vi "GetSystemSerialNumber.vi"(0 "VISA resource name":refnum<visa-resource-name>="COM5", 11 "error in (no error)":errorcluster, 12 "Open Serial":bool, 14 "Close Serial":bool) -> (3 "S/N":string="0", 4 "VISA resource name out":refnum<visa-resource-name>="COM5", 15 "error out":errorcluster)   [LabVIEW 2018]
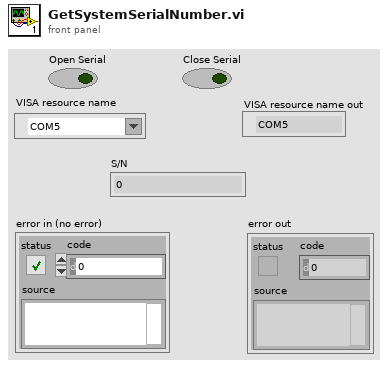
[diagram p1: front panel]
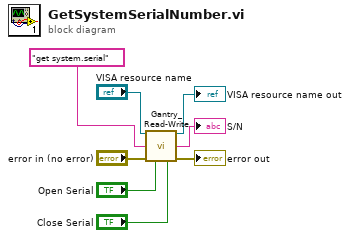
[diagram p0: block diagram]
diagram:
  n1 = call "Gantry_Read-Write.vi"("VISA resource name"="VISA resource name", "Command"="get system.serial", "error in (no error)"="error in (no error)", "Open Serial"="Open Serial", "Close Serial"="Close Serial") -> ("VISA resource name out"=→"VISA resource name out":refnum<visa-resource-name>, "Data"=→"S/N":string, "error out"=→"error out":errorcluster)  [unwired: 4 in, 4 out]
